vi "Z6_Beamline.set start page.vi"(0 "i ref in":refnum<vi>, 2 "Tab Control":refnum<vi>, 5 "error in (no error)":errorcluster) -> (14 "i ref out":refnum<vi>, 19 "error out":errorcluster)   [LabVIEW 2014, in "Z6_Beamline.lvlib"]
uses:
  Z6_Beamline.lvlib
  CSCore/CSSystem/CSSystemLib/CSSystemLib.lvlib
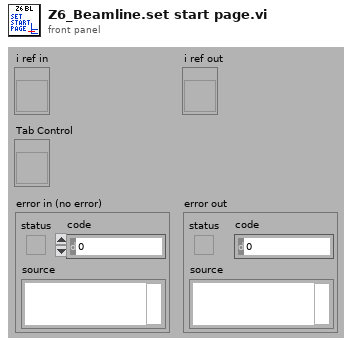
[diagram p1: front panel]
types:
  T1 = enum32{"PHELIX", "Northtower", "Southtower", "100TW COS"}
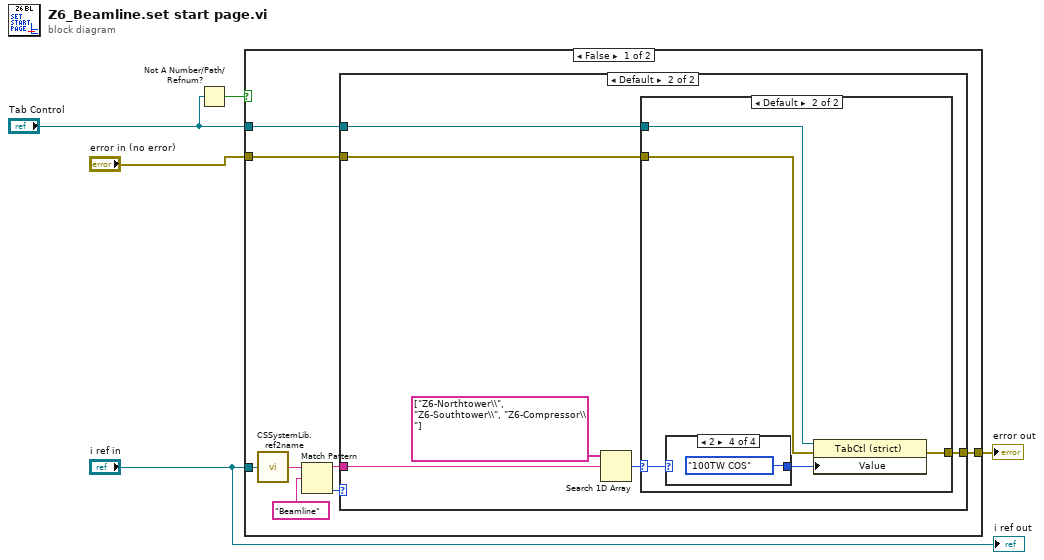
[diagram p0: block diagram]
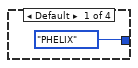
[diagram p4: hidden frame]
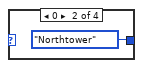
[diagram p5: hidden frame]
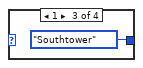
[diagram p6: hidden frame]
diagram:
  n1 = Not A Number/Path/Refnum?(number/path/refnum="Tab Control") -> (NaN/Path/Refnum?=w2:bool)
  n2 = case shown="False" w2 {
    tunnel: "i ref in" -> [w13 _]
    tunnel: "Tab Control" -> [w8 _]
    tunnel: [w7 w31] -> w4
    tunnel: "error in (no error)" -> [w6 w31]
    frame False {
      n3 = call "CSSystemLib.ref2name.vi"("obj refnum"=w13) -> ("name"=w9:string)
      n4 = Match Pattern(string=w9, regular expression="Beamline") -> (before substring=w11:string, offset past match=w12:i32)  [unwired: 1 in, 2 out]
      n5 = case shown="Default" w12 {
        tunnel: w11 -> [_ w15]
        tunnel: w8 -> [_ w18]
        tunnel: [w14 w17] -> w7
        tunnel: w6 -> [w14 w16]
        frame -1 {
        }
        frame Default {
          n6 = Search 1D Array(1D array=string[] ["Z6-Northtower\\", "Z6-Southtower\\", "Z6-Compressor\\"], element=w15) -> (index of element=w19:i32)  [unwired: 1 in]
          n7 = case shown="Default" w19 {
            selector: w19 -> [_ w23]
            tunnel: w18 -> [_ w26]
            tunnel: [w21 w25] -> w17
            tunnel: w16 -> [w21 w24]
            frame -1 {
            }
            frame Default {
              n8 = case shown="2" w23 {
                tunnel: [T1."PHELIX" ("Value") T1."Northtower" ("Value") T1."Southtower" ("Value") T1."100TW COS" ("Value")] -> w22
                frame Default {
                }
                frame 0 {
                }
                frame 1 {
                }
                frame 2 {
                }
              }
              n9 = property on="Property Node" class="TabCtl (strict)"(reference=w26, error in=w24, "Value"=w22) -> (error out=w25:errorcluster)  [unwired: 1 out]
            }
          }
        }
      }
    }
    frame True {
    }
  }
  "error out" <- w4
  "i ref out" <- "i ref in"
